vi "copyScriptToRunDir.vi"(8 "error in (no error)":errorcluster, 10 "Path in":path, 11 "FileNeologist in":refnum<class "FileNeologist.lvclass">) -> (0 "error out":errorcluster, 2 "Path out":path, 3 "FileNeologist out":refnum<class "FileNeologist.lvclass">)   [LabVIEW 2009, in "Tools.lvlib" / "Filing.lvlib" / "FileNeologist.lvclass"]
uses:
  FileNeologist.lvclass
  FileNeologist.lvclass/FileNeologist.ctl
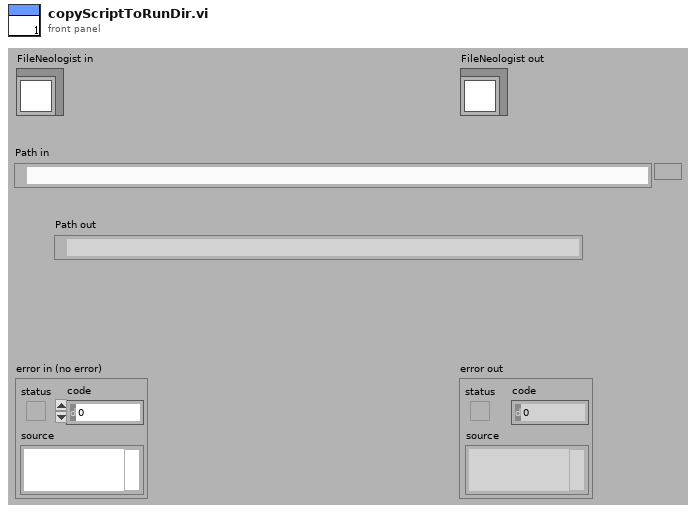
[diagram p1: front panel]
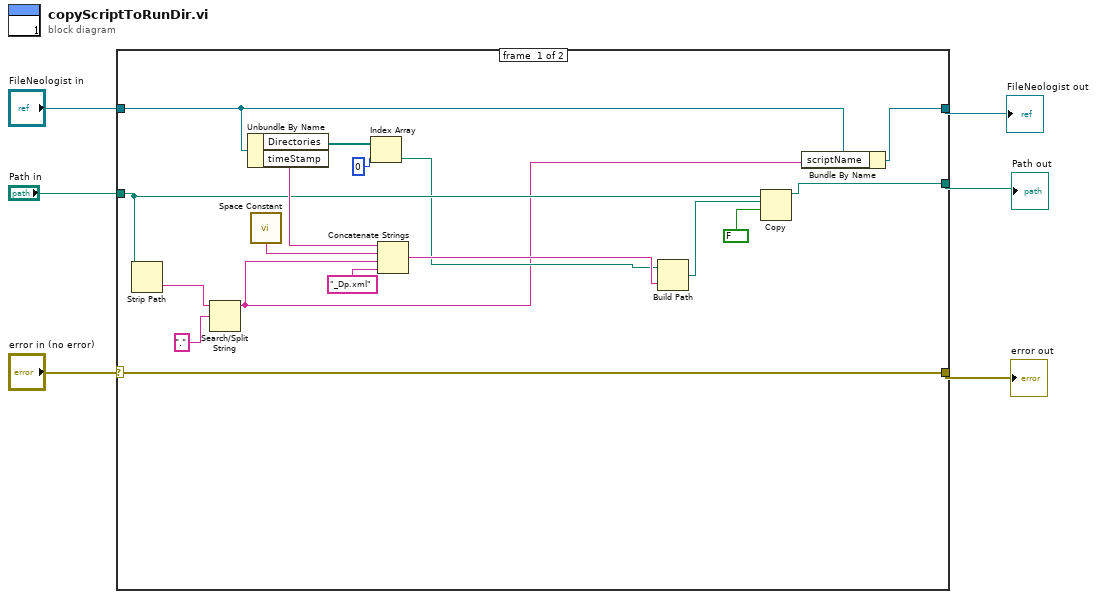
[diagram p0: block diagram]
diagram:
  n1 = case shown="No Error" "error in (no error)" {
    selector: "error in (no error)" -> [w10 w25]
    tunnel: [w10 w25] -> w5
    tunnel: [w13 w24] -> w3
    tunnel: "FileNeologist in" -> [w14 w24]
    tunnel: "Path in" -> [w18 _]
    tunnel: [w17 _] -> w1
    frame #0 {
      n2 = Strip Path(path=w18) -> (name=w7:string)  [unwired: 1 out]
      n3 = Search/Split String(string=w7, search string/char (-)=".") -> (substring before match=w8:string)  [unwired: 1 in, 2 out]
      n4 = Unbundle By Name(w14) -> ("Directories"=w16:path[], "timeStamp"=w19:string)
      n5 = call <vilib>:"Space Constant.vi"() -> ("String"=w21:string)
      n6 = Index Array(array=w16, index=0) -> (element=w11:path)
      n7 = Concatenate Strings(w19, w21, w8, "_Dp.xml") -> (w15:string)
      n8 = Build Path(base path=w11, name or relative path=w15) -> (appended path=w20:path)
      n9 = Copy(9:FALSE, 10:w20, 11:w18) -> (3:w17:path)  [unwired: 2 in, 2 out]
      n10 = Bundle By Name(cluster=w14, "scriptName"=w8) -> (w13:refnum<class "FileNeologist.lvclass">)
    }
    frame #1 {
    }
  }
  "error out" <- w5
  "FileNeologist out" <- w3
  "Path out" <- w1
